vi "rotate 2D array V4.vi"(9 "rotate y":i32=1, 10 "rotate x":i32, 11 "array in":cdb[][](array[numeric])=[[0.0+0.0i, 1.0+0.0i, 2.0+0.0i, 3.0+0.0i], [4.0+0.0i, 0.0+0.0i, 0.0+0.0i, 0.0+0.0i], [8.0+0.0i, 0.0+0.0i, 0.0+0.0i, 0.0+0.0i], [13.0+0.0i, 0.0+0.0i, 99.0+0.0i, 0.0+0.0i]]) -> (3 "array out":cdb[][](array[numeric])=[[13.0+0.0i, 0.0+0.0i, 99.0+0.0i, 0.0+0.0i], [0.0+0.0i, 1.0+0.0i, 2.0+0.0i, 3.0+0.0i], [4.0+0.0i, 0.0+0.0i, 0.0+0.0i, 0.0+0.0i], [8.0+0.0i, 0.0+0.0i, 0.0+0.0i, 0.0+0.0i]])   [LabVIEW 2010]
doc: "size has to be a prime number"
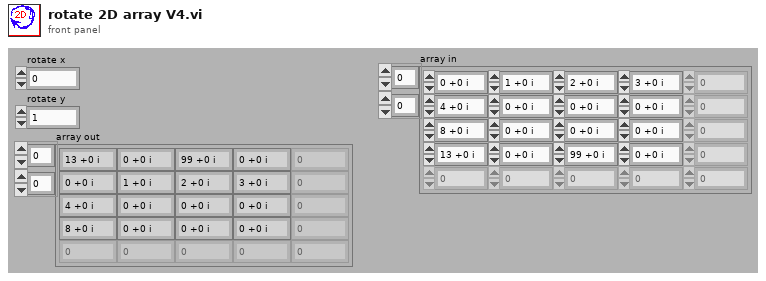
[diagram p1: front panel]
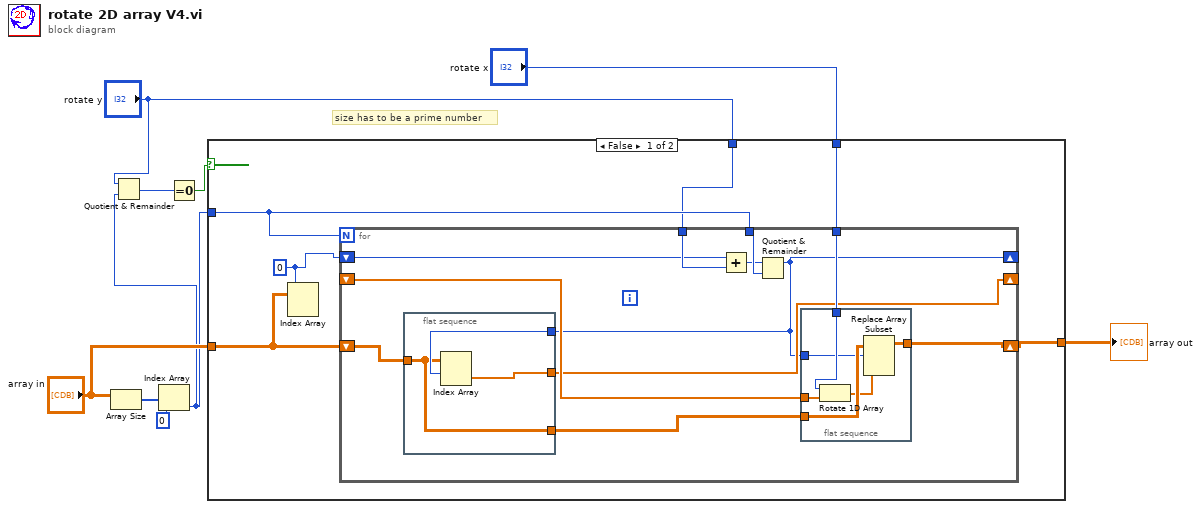
[diagram p0: block diagram]
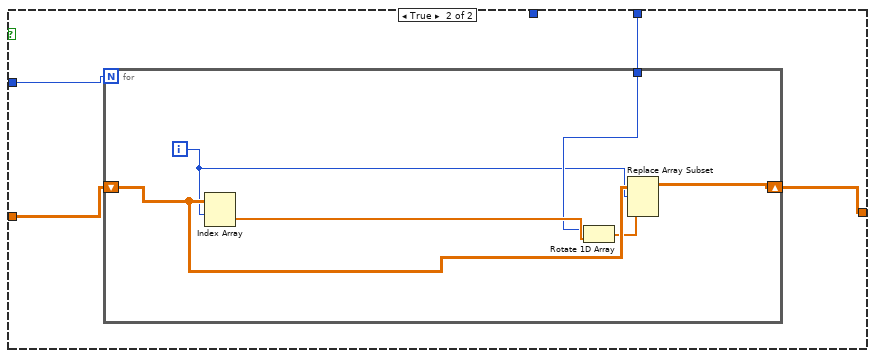
[diagram p2: hidden frame]
diagram:
  # "size has to be a prime number"
  n1 = Array Size(array="array in") -> (size(s)=w8:i32[])
  n2 = Index Array(array=w8, index=0) -> (element=w3:i32)
  n3 = Quotient & Remainder(x="rotate y", y=w3) -> (x-y*floor(x/y)=w2:i32)  [unwired: 1 out]
  n4 = Equal To 0?(x=w2) -> (x = 0?=w1:bool)
  n5 = case shown="False" w1 {
    tunnel: "array in" -> [w11 w39]
    tunnel: "rotate x" -> [w15 w38]
    tunnel: [w14 w37] -> w5
    tunnel: w3 -> [w13 w36]
    tunnel: "rotate y" -> [w12 _]
    frame False {
      w10 = 0 ("index")
      n6 = Index Array(array=w11, index (row)=w10) -> ()  [unwired: 1 in, 1 out]
      n7 = for {
        N: w13 -> [_]
        tunnel: w13 -> [w26]
        shift-right: [w18] -> _
        shift-left: _ -> [w19]
        tunnel: w12 -> [w24]
        tunnel: w15 -> [w23]
        shift-right: [w22] -> w14
        shift-left: w11 -> [w21]
        shift-right: [w17] -> _
        shift-left: w10 -> [w20]
        n8 = flat-sequence {
          tunnel: w21 -> [w34]
          tunnel: [w33] -> w18
          tunnel: w17 -> [w35]
          tunnel: [w34] -> w16
          frame #0 {
            n9 = Index Array(array=w34, index (row)=w35) -> (element=w33:cdb[])  [unwired: 1 in]
          }
        }
        n10 = Add(x=w20, y=w24) -> (x+y=w25:i32)
        n11 = Quotient & Remainder(x=w25, y=w26) -> (x-y*floor(x/y)=w17:i32)  [unwired: 1 out]
        n12 = flat-sequence {
          tunnel: w23 -> [w32]
          tunnel: [w31] -> w22
          tunnel: w16 -> [w30]
          tunnel: w19 -> [w28]
          tunnel: w17 -> [w27]
          frame #0 {
            n13 = Rotate 1D Array(1:w28, 2:w32) -> (0:w29:cdb[])
            n14 = Replace Array Subset(array=w30, new element=w29, index (row)=w27) -> (w31:cdb[][])  [unwired: 1 in]
          }
        }
      }
    }
    frame True {
      n15 = for {
        N: w36 -> [_]
        shift-right: [w45] -> w37
        shift-left: w39 -> [w44]
        tunnel: w38 -> [w41]
        i -> [w40]
        n16 = Index Array(array=w44, index (row)=w40) -> (element=w42:cdb[])  [unwired: 1 in]
        n17 = Rotate 1D Array(1:w42, 2:w41) -> (0:w43:cdb[])
        n18 = Replace Array Subset(array=w44, new element=w43, index (row)=w40) -> (w45:cdb[][])  [unwired: 1 in]
      }
    }
  }
  "array out" <- w5
